vi "Финал.vi"() -> ()   [LabVIEW 2017]
panel:
  in  "Reset":bool
  in  "C":bool
  in  "Exec":bool
  out "Result":T1
  out "FLAGS":T2
  in  "Func":T3
  in  "B":T4
  in  "A":T5
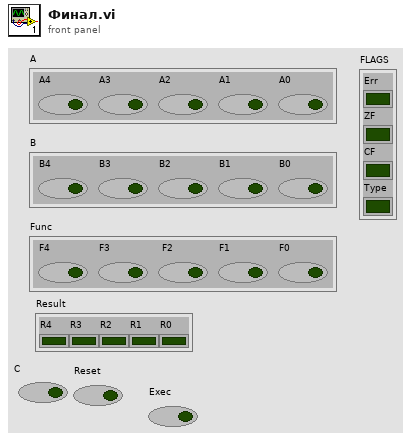
[diagram p1: front panel]
types:
  T1 = cluster{"R4":bool, "R3":bool, "R2":bool, "R1":bool, "R0":bool}
  T2 = cluster{"Err":bool, "ZF":bool, "CF":bool, "Type":bool}
  T3 = cluster{"F4":bool, "F3":bool, "F2":bool, "F1":bool, "F0":bool}
  T4 = cluster{"B4":bool, "B3":bool, "B2":bool, "B1":bool, "B0":bool}
  T5 = cluster{"A4":bool, "A3":bool, "A2":bool, "A1":bool, "A0":bool}
  T6 = cluster{"Q4":bool, "Q33QQq3Q3Q3Q3Q3Q3Q3Q":bool, "Q2":bool, "Q1`":bool, "Q0":bool}
  T7 = cluster{"Err":bool, "CF":bool, "ZF":bool, "Type":bool}
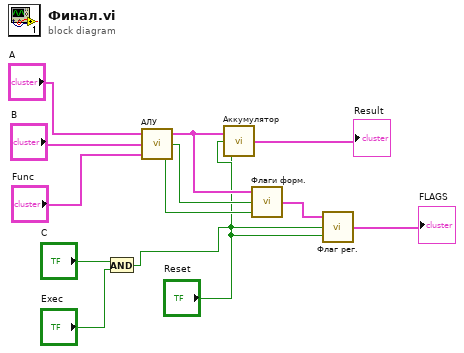
[diagram p0: block diagram]
diagram:
  n1 = And(x="C", y="Exec") -> (x .and. y?=w1:bool)
  n2 = call "АЛУ.vi"("Func"="Func", "B"="B", "A"="A") -> ("Type"=w6:bool, "C"=w7:bool, "Result"=w8:T1)
  n3 = call "Аккумулятор.vi"("С"=w1, "Reset"="Reset", "Cluster"=w8) -> ("Q"=→"Result":T6)
  n4 = call "Флаги форм..vi"("Type"=w6, "C"=w7, "R"=w8) -> ("FLAGS"=w5:T2)
  n5 = call "Флаг рег..vi"("Reset"="Reset", "C"=w1, "Enter"=w5) -> ("Exit"=→"FLAGS":T7)
